vi "AddIRSEQ.vi"(0 "VISA resource name":refnum<visa-resource-name>, 1 "Test Voltage (V)":string, 2 "Pre-Check Delay (s)":string, 3 "Dwell Time (s)":string, 4 "Min IR Limit (ohm)":string, 5 "Max IR Limit (ohm)":string, 7 "error in (no error)":errorcluster, 8 "Sequence Number":string, 9 "DUT Type I":string(combo)="Isolated DUT", 10 "Sequence Name":string, 11 "DUT Type II (DCW Only)":string(combo)="Resistive DUT") -> (20 "VISA resource name out":refnum<visa-resource-name>, 25 "Error Message":string, 26 "Error Code":i32, 27 "error out":errorcluster)   [LabVIEW 2010, in "VITREK V7X.lvlib"]
doc: "Add a new IR test step into a sequence and save this sequence into the requested store number."
uses:
  VITREK V7X.lvlib
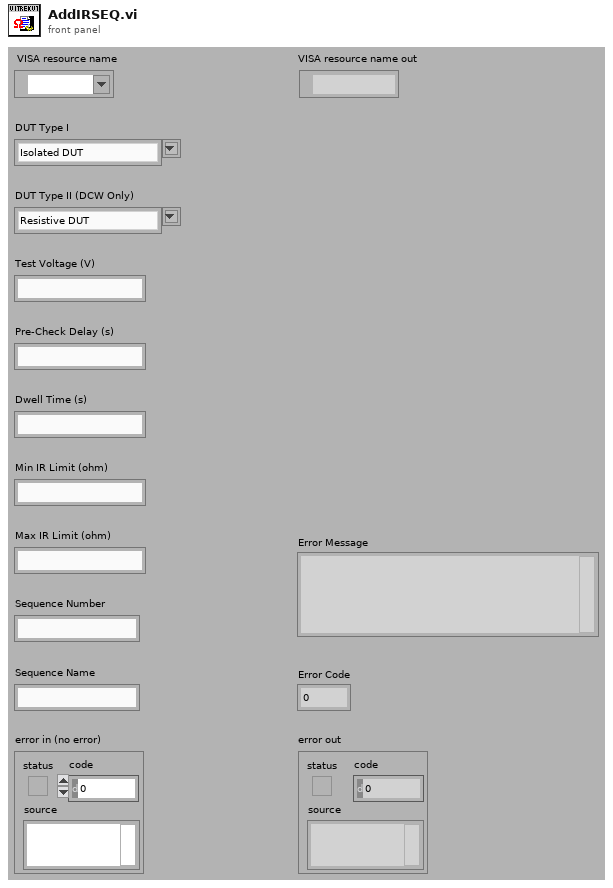
[diagram p1: front panel]
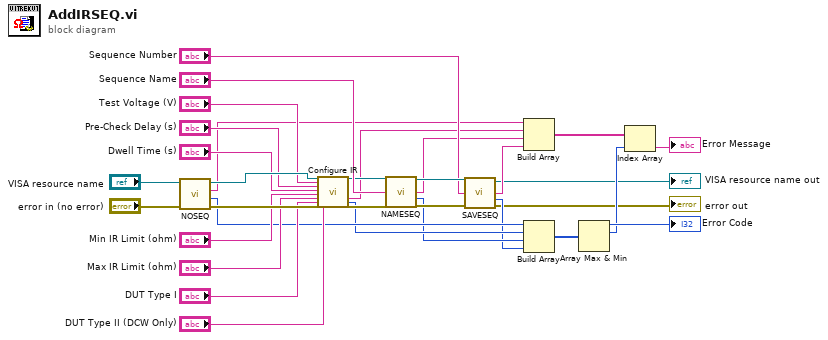
[diagram p0: block diagram]
diagram:
  n1 = call "NOSEQ.vi"("error in (no error)"="error in (no error)", "VISA resource name"="VISA resource name") -> ("error out"=w24:errorcluster, "Error Code"=w7:i32, "Error Message"=w15:string, "VISA resource name out"=w26:refnum<visa-resource-name>)  [unwired: 6 in]
  n2 = call "Configure IR.vi"("VISA resource name"=w26, "Test Voltage (V)"="Test Voltage (V)", "Pre-Check Delay (s)"="Pre-Check Delay (s)", "Dwell Time (s)"="Dwell Time (s)", "Min IR Limit (ohm)"="Min IR Limit (ohm)", "Max IR Limit (ohm)"="Max IR Limit (ohm)", "DUT Type I"="DUT Type I", "error in (no error)"=w24, "DUT Type II"="DUT Type II (DCW Only)") -> ("VISA resource name out"=w25:refnum<visa-resource-name>, "Error Message"=w14:string, "Error Code"=w6:i32, "error out"=w23:errorcluster)  [unwired: 14 in, 1 out]
  n3 = call "NAMESEQ.vi"("VISA resource name"=w25, "Sequence Name"="Sequence Name", "error in (no error)"=w23) -> ("VISA resource name out"=w29:refnum<visa-resource-name>, "Error Message"=w13:string, "Error Code"=w5:i32, "error out"=w30:errorcluster)  [unwired: 9 in]
  n4 = call "SAVESEQ.vi"("VISA resource name"=w29, "Sequence Number"="Sequence Number", "error in (no error)"=w30) -> ("VISA resource name out"=→"VISA resource name out":refnum<visa-resource-name>, "Error Message"=w12:string, "Error Code"=w4:i32, "error out"=→"error out":errorcluster)  [unwired: 9 in]
  n5 = Build Array(w15, w14, w13, w12) -> (w11:string[])
  n6 = Build Array(w7, w6, w5, w4) -> (w9:i32[])
  n7 = Array Max & Min(array=w9) -> (max value=→"Error Code":i32, max index (indices)=w3:i32)  [unwired: 2 out]
  n8 = Index Array(array=w11, index=w3) -> (element=→"Error Message":string)
